vi "feet to milliseconds.vi"(11 "Distance in feet wanted":dbl) -> (3 "milliseconds":dbl)   [LabVIEW 2017]
panel:
  # "Doesn't do anything right now"
  # "Actually, it does"
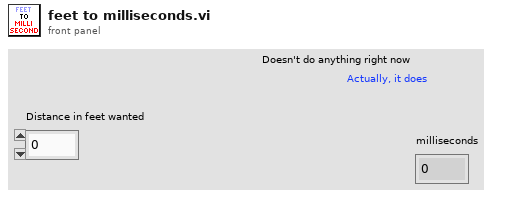
[diagram p1: front panel]
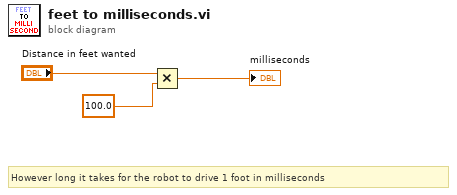
[diagram p0: block diagram]
diagram:
  # "However long it takes for the robot to drive 1 foot in milliseconds"
  n1 = Multiply(x="Distance in feet wanted", y=100.0) -> (x*y=→"milliseconds":dbl)
